vi "auto_alignment_v2.vi"(0 "meter-visa":refnum<visa-resource-name>, 1 "xStart":dbl=264.0 format="%#_13g", 2 "yStart":dbl=123.0 format="%#_13g", 3 "NM-params":T1={"alpha"=1.0, "gamma"=2.0, "rho"=0.5, "sigma"=0.5, "simplex L"=0.5}, 5 "PD Values":cluster{"PD1":dbl, "PD2":dbl, "PD3":dbl}, 6 "F=cRIO":bool, 7 "stage-refs":T2, 9 "meter-error-in":errorcluster, 11 "stage-error-in":errorcluster, 12 "trial #":i32, 13 "path-in":path=path "C:/Users/hpDIRC/Desktop/Tyler/t3.csv") -> (4 "Optimized Location":dbl[](array[numeric]), 8 "squared_error":dbl, 10 "meter-error-out":errorcluster, 14 "run time (min)":dbl, 15 "stage-error-out":errorcluster)   [LabVIEW 2024]
uses:
  O:/DSG/Tyler/EIC/DIRC/daq/automated/Thorlabs.MotionControl.IntegratedStepperMotorsCLI.dll
  Thorlabs.MotionControl.IntegratedStepperMotorsCLI.dll
  O:/DSG/Tyler/EIC/DIRC/daq/automated/Thorlabs.MotionControl.Benchtop.StepperMotorCLI.dll
  Thorlabs.MotionControl.Benchtop.StepperMotorCLI.dll
  5b59031f-b1ff-41af-80a7-e72a33ebffa1.vi
  <vilib>/Array/Sort 2D Array - Pop Stack.vi
  <vilib>/Array/Sort 2D Array - Push Stack.vi
  5b59031f-b1ff-41af-80a7-e72a33ebffa1.vi/269d4b3b-47f5-49e3-8884-44851e4dd9d5.vi
  5b59031f-b1ff-41af-80a7-e72a33ebffa1.vi/6d99389c-673d-4efb-bf33-19b32bcf4cf8.vi
  <vilib>/Analysis/NI_AALBase.lvlib
panel:
  in  "nSamples":dbl=10.0 caption="# Samples"
  in  "simplex-limit":dbl=1e-06 caption="Simplex Length Convergence Goal" format="%#_13g"
  in  "value-limit":dbl=0.04 caption="Value Convergence Goal" format="%#_13g"
  out "Pts Tested":dbl[][](array[numeric])
  out "x_c":dbl[](array[numeric])
  out "x_e":dbl[](array[numeric])
  out "x_r":dbl[](array[numeric])
  out "x_o":dbl[](array[numeric])
  out "iterations timeout":bool
  out "simplex converge":bool
  out "value converge":bool
  out "simplex leg lengths":dbl[](array[numeric])
  in  "stop":bool
  # "centroid"
  # "reflection point"
  # "expansion point"
  # "contraction point"
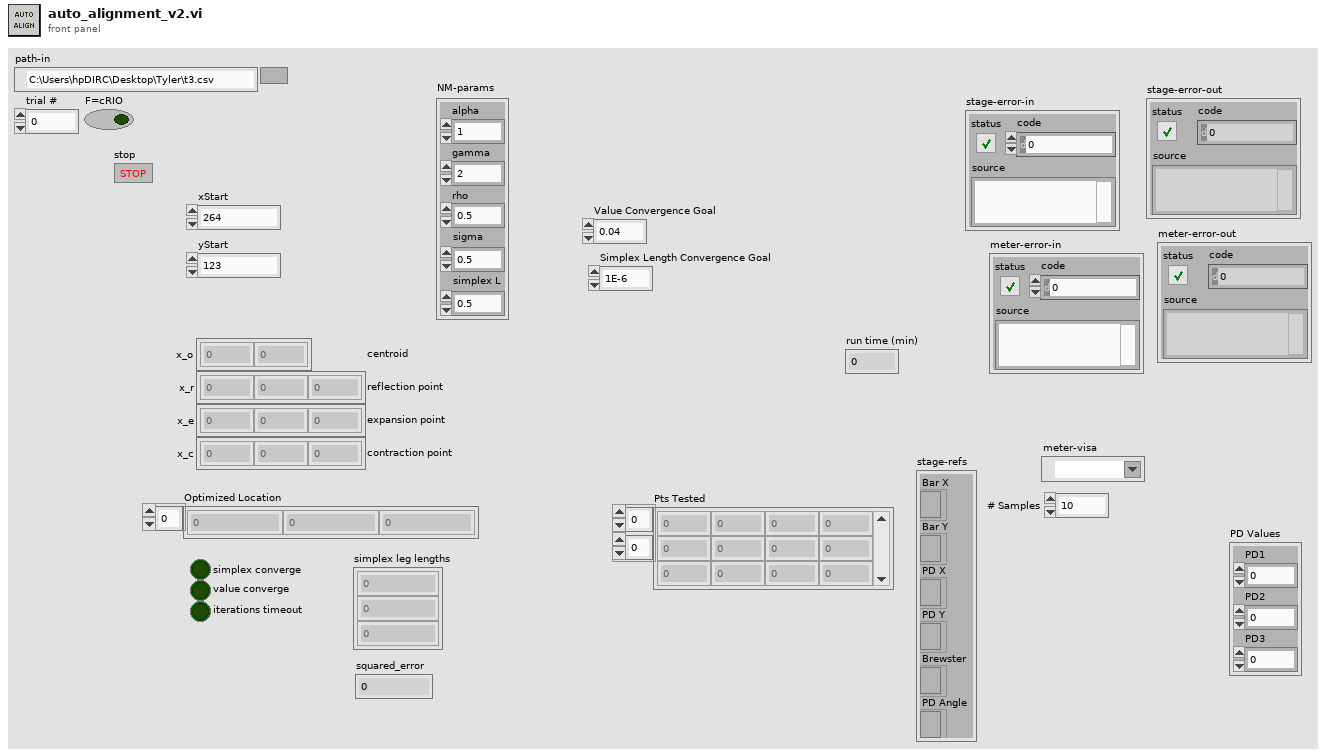
[diagram p1: front panel]
types:
  T1 = cluster{"alpha":dbl, "gamma":dbl, "rho":dbl, "sigma":dbl, "simplex L":dbl}
  T2 = cluster{"Bar X":refnum<k24>, "Bar Y":refnum<k24>, "PD X":refnum<k24>, "PD Y":refnum<k24>, "Brewster":refnum<k24>, "PD Angle":refnum<k24>}
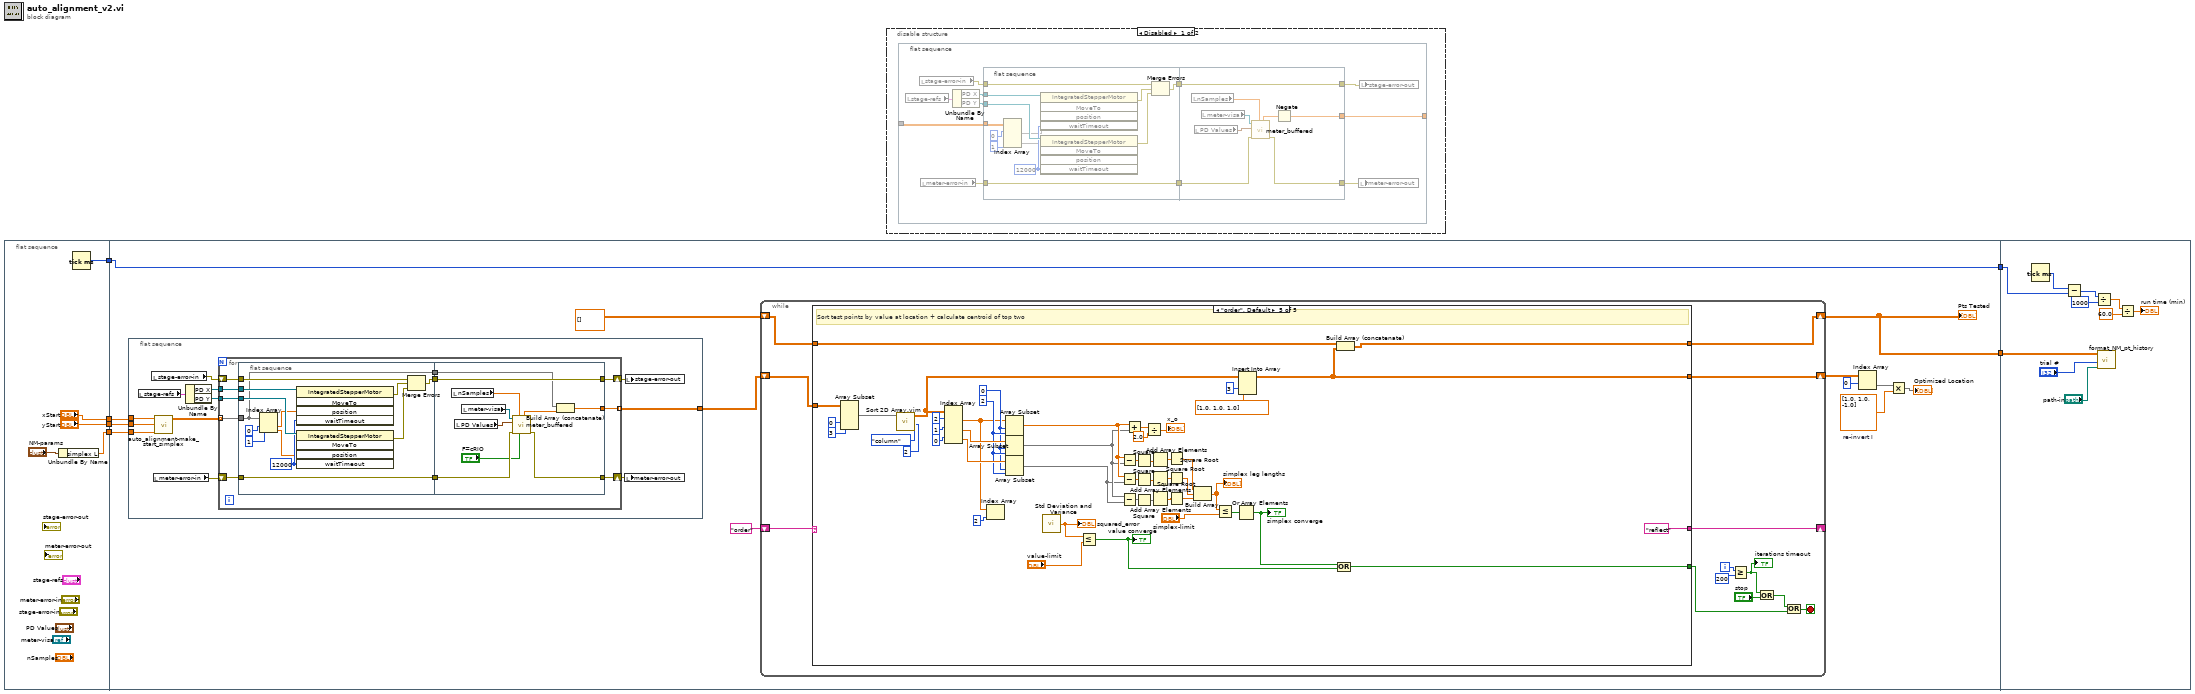
[diagram p0: block diagram]
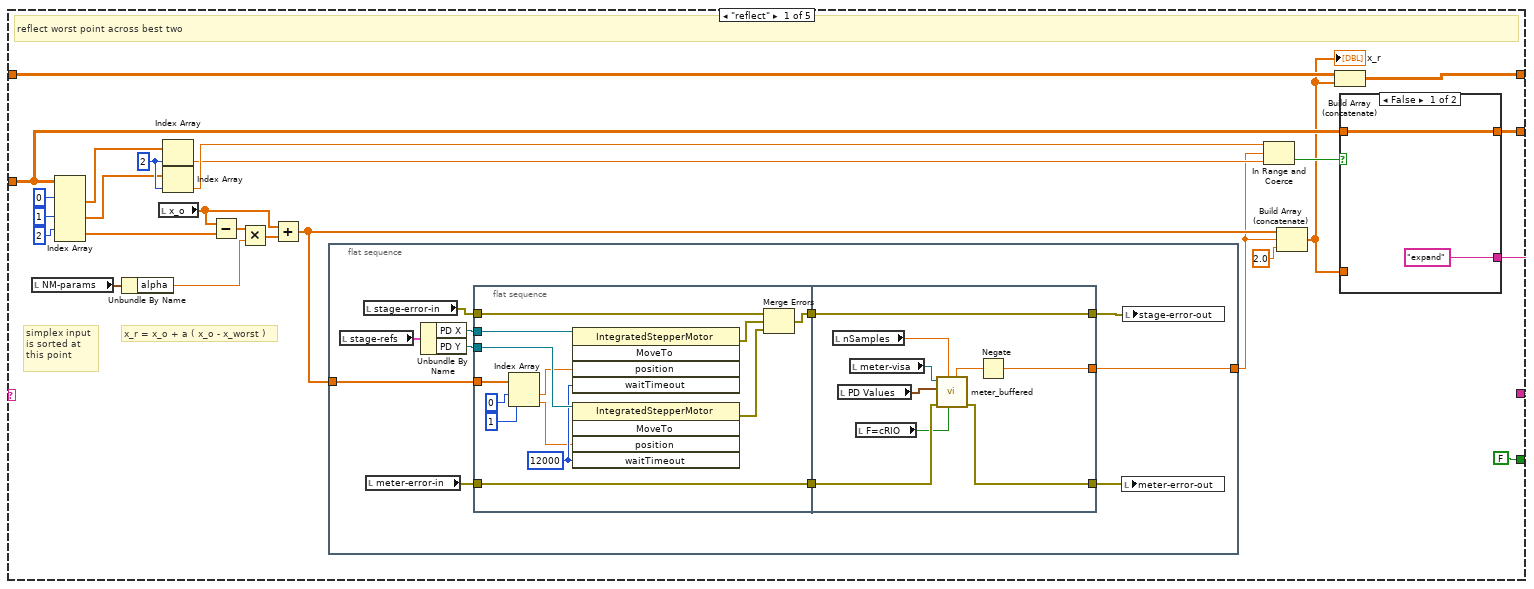
[diagram p3: hidden frame]
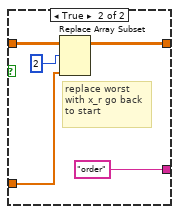
[diagram p4: hidden frame]
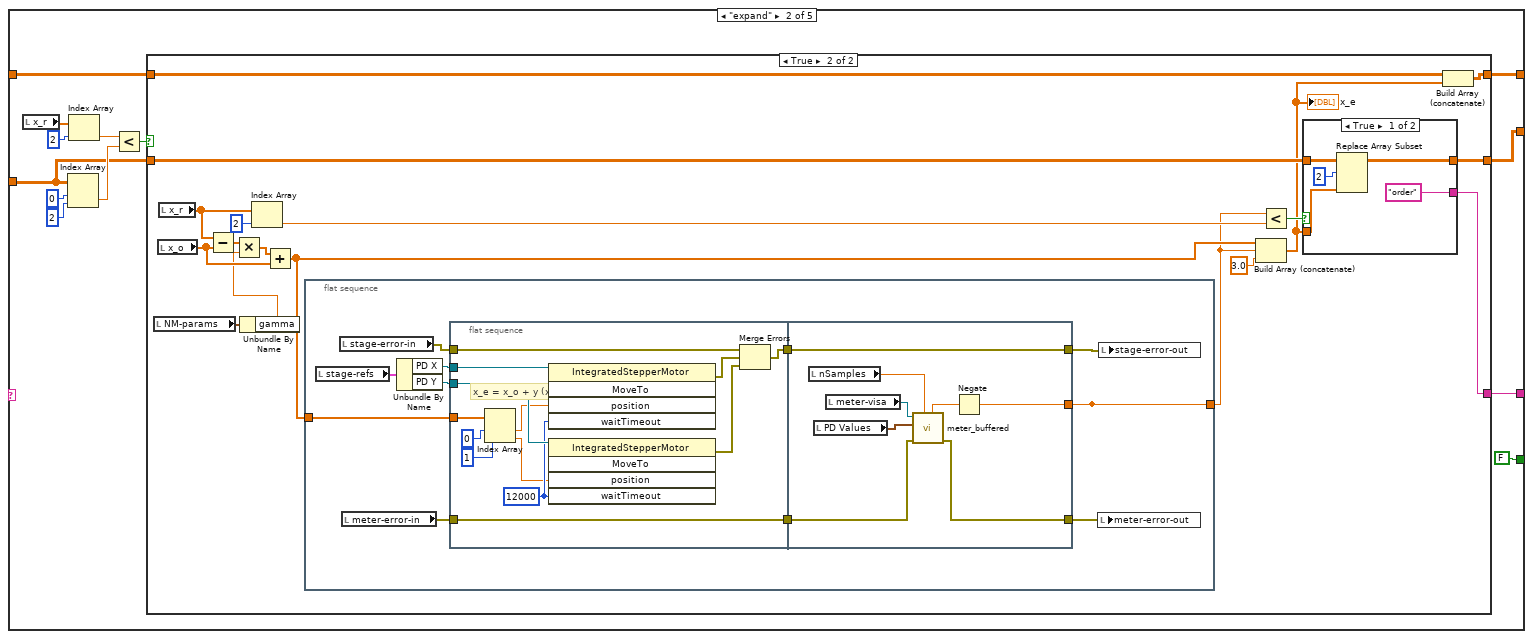
[diagram p5: hidden frame]
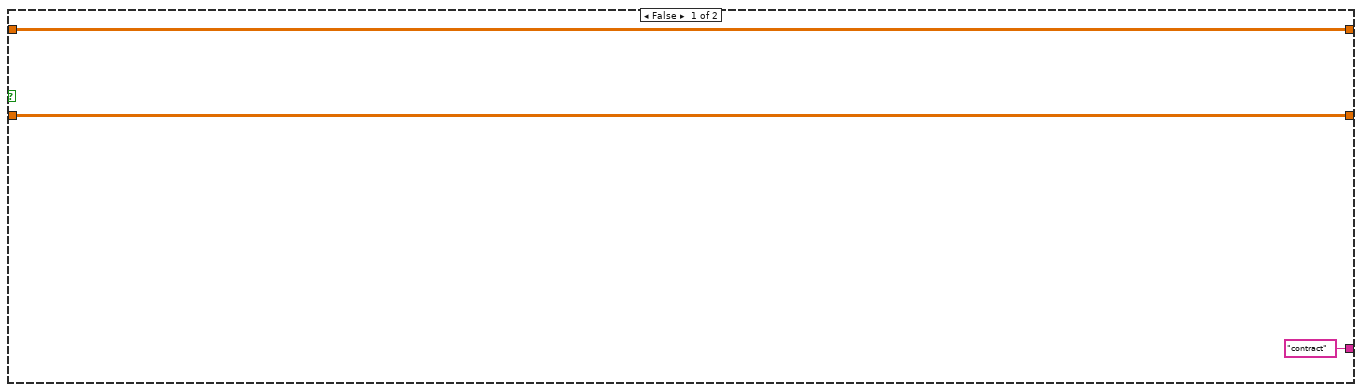
[diagram p6: hidden frame]
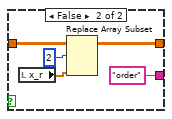
[diagram p7: hidden frame]
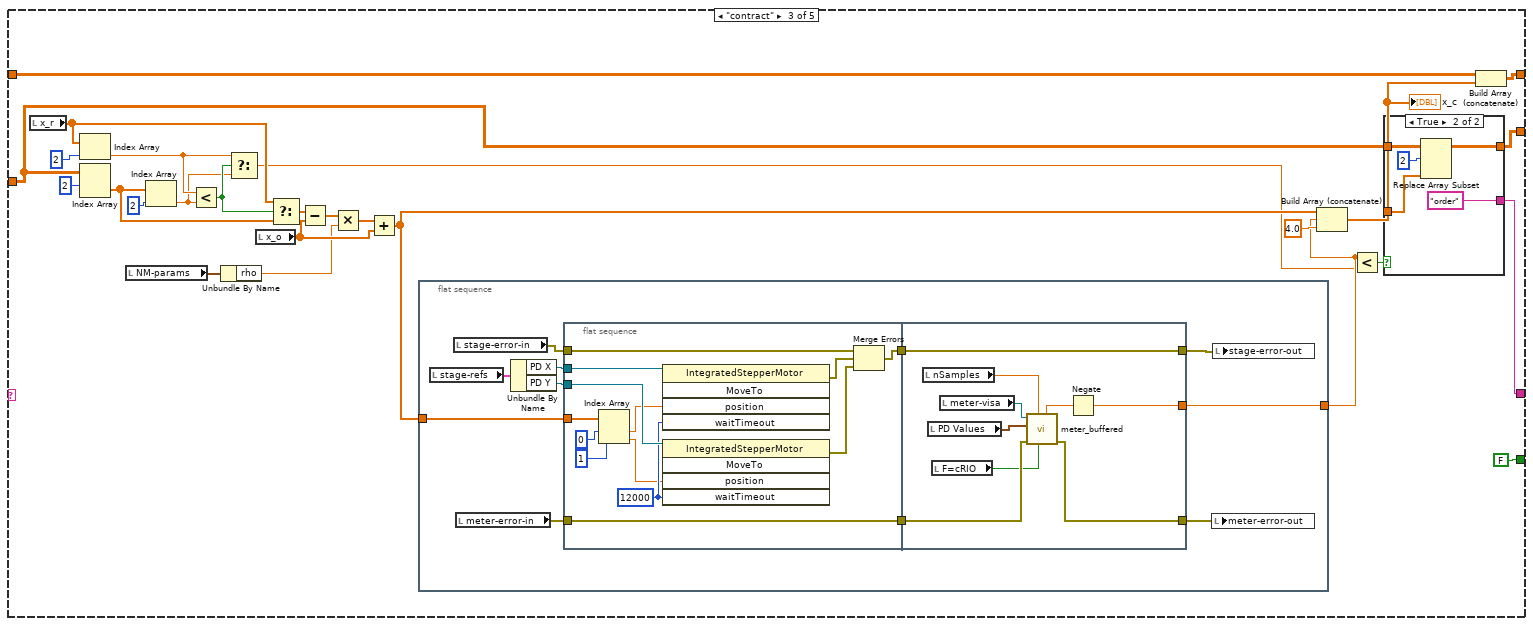
[diagram p8: hidden frame]
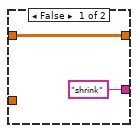
[diagram p9: hidden frame]
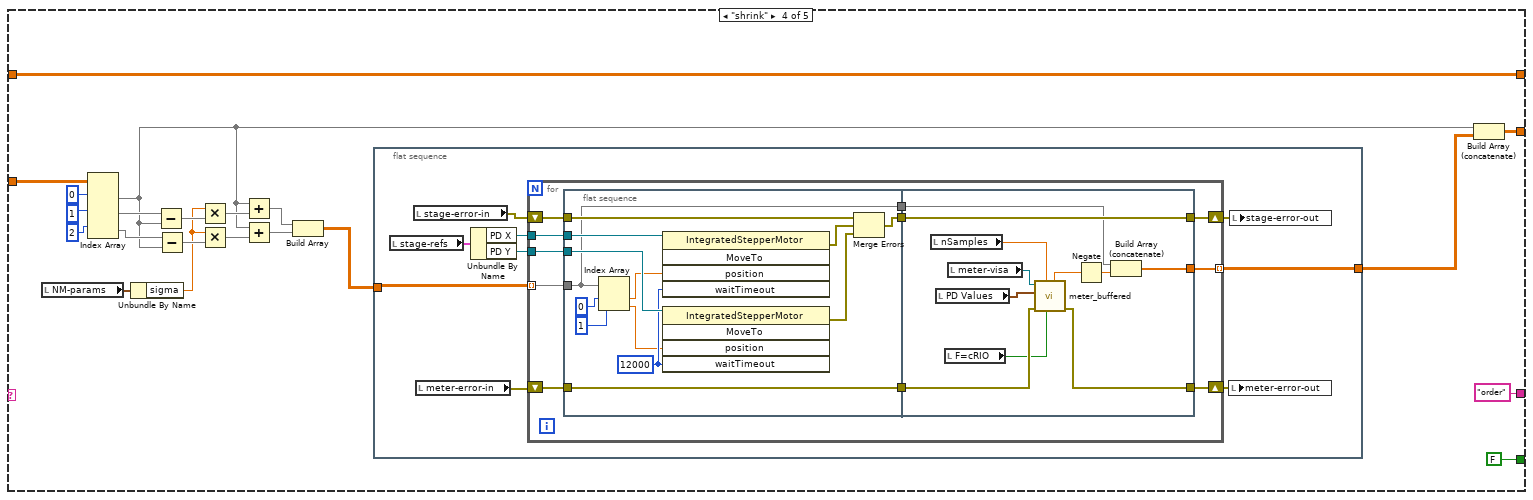
[diagram p10: hidden frame]
diagram:
  n1 = flat-sequence {
    tunnel: [w11] -> w5
    tunnel: ["yStart"] -> w3
    tunnel: ["xStart"] -> w2
    tunnel: [w7] -> w1
    tunnel: [w22] -> w6
    tunnel: w5 -> [w21]
    tunnel: [w21] -> w4
    tunnel: w3 -> [w13]
    tunnel: w2 -> [w14]
    tunnel: w1 -> [w12]
    tunnel: w6 -> [w411]
    tunnel: w4 -> [w409]
    frame #0 {
      n2 = Unbundle By Name("NM-params") -> ("simplex L"=w7:dbl)
      n3 = Tick Count (ms)() -> (millisecond timer value=w11:u32)
    }
    frame #1 {
      w16 = dbl[] [1.0, 1.0, -1.0]  # re-invert I
      n4 = flat-sequence {
        tunnel: [w33] -> w15
        tunnel: w13 -> [w32]
        tunnel: w14 -> [w31]
        tunnel: w12 -> [w25]
        frame #0 {
          n5 = local read "stage-refs"() -> (w27:T2)
          n6 = local read "stage-error-in"() -> (w28:errorcluster)
          n7 = local read "meter-error-in"() -> (w26:errorcluster)
          n8 = call "auto_alignment-make_start_simplex.vi"("L"=w25, "yStart"=w32, "xStart"=w31) -> ("Array"=w34:dbl[][])  [unwired: 8 in]
          n9 = Unbundle By Name(w27) -> ("PD X"=w36:refnum<k24>, "PD Y"=w35:refnum<k24>)
          n10 = for {
            tunnel: w36 -> [w47]
            tunnel: w35 -> [w46]
            tunnel: w34 -> [w43] mode=indexing
            shift-right: [w41] -> w29
            shift-left: w28 -> [w45]
            tunnel: [w44] -> w33 mode=indexing
            shift-right: [w42] -> w30
            shift-left: w26 -> [w40]
            n11 = flat-sequence {
              tunnel: w47 -> [w58]
              tunnel: w46 -> [w57]
              tunnel: w45 -> [w51]
              tunnel: w43 -> [w49]
              tunnel: w40 -> [w48]
              tunnel: [w50] -> w39
              tunnel: [w49] -> w38
              tunnel: [w48] -> w37
              tunnel: [w70] -> w41
              tunnel: [w66] -> w42
              tunnel: [w69] -> w44
              tunnel: w39 -> [w70]
              tunnel: w38 -> [w68]
              tunnel: w37 -> [w67]
              frame #0 {
                w56 = 12000 ("waitTimeout")
                n12 = Index Array(array=w49, index #1=0 ("index"), index #2=1 ("index")) -> (element #1=w53:dbl, element #2=w52:dbl)
                n13 = invoke class="IntegratedStepperMotor" method="MoveTo"(reference=w58, "position"=w53, "waitTimeout"=w56) -> (error out=w60:errorcluster)  [unwired: 2 in, 4 out]
                n14 = invoke class="IntegratedStepperMotor" method="MoveTo"(reference=w57, "position"=w52, "waitTimeout"=w56) -> (error out=w59:errorcluster)  [unwired: 2 in, 4 out]
                n15 = Merge Errors(w51, w60, w59) -> (w50:errorcluster)
              }
              frame #1 {
                n16 = local read "nSamples"() -> (w65:dbl)
                n17 = local read "PD Values"() -> (w63:cluster{"PD1":dbl, "PD2":dbl, "PD3":dbl})
                n18 = local read "meter-visa"() -> (w64:refnum<visa-resource-name>)
                n19 = call "meter_buffered.vi"("F=cRIO"="F=cRIO", "Samples"=w65, "error in"=w67, "PD ranges"=w63, "meter-VISA"=w64) -> ("error out"=w66:errorcluster, "iCorr"=w61:dbl)  [unwired: 2 in, 3 out]
                n20 = Build Array (concatenate)(w68, w61) -> (w69:dbl[])
              }
            }
          }
          n21 = local write "meter-error-out"(w30) -> ()
          n22 = local write "stage-error-out"(w29) -> ()
        }
      }
      n23 = while {
        shift-right: [w81] -> w20
        shift-left: w15 -> [w80]
        shift-right: [w82] -> _
        shift-left: "order" -> [w83]
        shift-right: [w78] -> w22
        shift-left: dbl[][] [] -> [w79]
        i -> [w74]
        stop <- w72 stop-if-true
        n24 = case shown="\"order\", Default" w83 {
          tunnel: w80 -> [w94 w154 w237 w310 w395]
          tunnel: [FALSE FALSE FALSE FALSE w376] -> w76
          tunnel: [w93 w153 w238 w299 w369] -> w81
          tunnel: [w95 w152 w239 "order" "reflect"] -> w82
          tunnel: w79 -> [w91 w150 w233 w297 w368]
          tunnel: [w90 w149 w232 w297 w373] -> w78
          frame "reflect" {
            w102 = 2 ("index")
            # "simplex input\nis sorted at\nthis point"
            # "x_r = x_o + a ( x_o - x_worst )"
            # "reflect worst point across best two"
            n25 = local read "NM-params"() -> (w85:T1)
            n26 = Index Array(array=w94, index (row) #1=0 ("index (row)"), index (row) #2=1 ("index (row)"), index (row) #3=2 ("index (row)")) -> (element #1=w101:dbl[], element #2=w100:dbl[], element #3=w103:dbl[])  [unwired: 3 in]
            n27 = Unbundle By Name(w85) -> ("alpha"=w84:dbl)
            n28 = local read "x_o"() -> (w96:dbl[])
            n29 = Index Array(array=w101, index=w102) -> (element=w98:dbl)
            n30 = Index Array(array=w100, index=w102) -> (element=w99:dbl)
            n31 = Subtract(x=w96, y=w103) -> (x-y=w107:dbl[])
            n32 = Multiply(x=w107, y=w84) -> (x*y=w106:dbl[])
            n33 = Add(x=w96, y=w106) -> (x+y=w87:dbl[])
            n34 = flat-sequence {
              tunnel: [w109] -> w86
              tunnel: w87 -> [w110]
              frame #0 {
                n35 = local read "stage-refs"() -> (w114:T2)
                n36 = local read "stage-error-in"() -> (w115:errorcluster)
                n37 = local read "meter-error-in"() -> (w113:errorcluster)
                n38 = Unbundle By Name(w114) -> ("PD X"=w119:refnum<k24>, "PD Y"=w118:refnum<k24>)
                n39 = flat-sequence {
                  tunnel: w119 -> [w130]
                  tunnel: w118 -> [w129]
                  tunnel: w115 -> [w123]
                  tunnel: w110 -> [w121]
                  tunnel: w113 -> [w120]
                  tunnel: [w122] -> w112
                  tunnel: [w120] -> w111
                  tunnel: [w141] -> w116
                  tunnel: [w138] -> w117
                  tunnel: [w134] -> w109
                  tunnel: w112 -> [w141]
                  tunnel: w111 -> [w139]
                  frame #0 {
                    w128 = 12000 ("waitTimeout")
                    n40 = Index Array(array=w121, index #1=0 ("index"), index #2=1 ("index")) -> (element #1=w125:dbl, element #2=w124:dbl)
                    n41 = invoke class="IntegratedStepperMotor" method="MoveTo"(reference=w130, "position"=w125, "waitTimeout"=w128) -> (error out=w132:errorcluster)  [unwired: 2 in, 4 out]
                    n42 = invoke class="IntegratedStepperMotor" method="MoveTo"(reference=w129, "position"=w124, "waitTimeout"=w128) -> (error out=w131:errorcluster)  [unwired: 2 in, 4 out]
                    n43 = Merge Errors(w123, w132, w131) -> (w122:errorcluster)
                  }
                  frame #1 {
                    n44 = local read "nSamples"() -> (w137:dbl)
                    n45 = local read "PD Values"() -> (w135:cluster{"PD1":dbl, "PD2":dbl, "PD3":dbl})
                    n46 = local read "meter-visa"() -> (w136:refnum<visa-resource-name>)
                    n47 = local read "F=cRIO"() -> (w133:bool)
                    n48 = call "meter_buffered.vi"("F=cRIO"=w133, "Samples"=w137, "error in"=w139, "PD ranges"=w135, "meter-VISA"=w136) -> ("error out"=w138:errorcluster, "iCorr"=w140:dbl)  [unwired: 2 in, 3 out]
                    n49 = Negate(x=w140) -> (-x=w134:dbl)
                  }
                }
                n50 = local write "meter-error-out"(w117) -> ()
                n51 = local write "stage-error-out"(w116) -> ()
              }
            }
            n52 = In Range and Coerce(upper limit=w99, x=w86, lower limit=w98) -> (In Range?=w97:bool)  [unwired: 1 out]
            n53 = Build Array (concatenate)(w87, w86, 2.0) -> (w89:dbl[])
            "x_r" <- w89
            n54 = Build Array (concatenate)(w91, w89) -> (w90:dbl[][])
            n55 = case shown="False" w97 {
              tunnel: ["expand" "order"] -> w95
              tunnel: w94 -> [w142 w148]
              tunnel: [w142 w145] -> w93
              tunnel: w89 -> [_ w146]
              frame False {
              }
              frame True {
                # "replace worst \nwith x_r go back\nto start"
                n56 = Replace Array Subset(array=w148, new element=w146, index (row)=2) -> (w145:dbl[][])  [unwired: 1 in]
              }
            }
          }
          frame "expand" {
            n57 = local read "x_r"() -> (w159:dbl[])
            n58 = Index Array(array=w154, index (row)=0, index (col)=2 ("disabled index (col)")) -> (element=w157:dbl)
            n59 = Index Array(array=w159, index=2) -> (element=w156:dbl)
            n60 = Less?(x=w156, y=w157) -> (x < y?=w155:bool)
            n61 = case shown="True" w155 {
              tunnel: w154 -> [w164 w175]
              tunnel: [w164 w174] -> w153
              tunnel: ["contract" w173] -> w152
              tunnel: w150 -> [w162 w172]
              tunnel: [w162 w171] -> w149
              frame False {
              }
              frame True {
                # "x_e = x_o + y (x _r - x _o)"
                n62 = local read "NM-params"() -> (w166:T1)
                n63 = local read "x_o"() -> (w180:dbl[])
                n64 = local read "x_r"() -> (w179:dbl[])
                n65 = Subtract(x=w179, y=w180) -> (x-y=w182:dbl[])
                n66 = Unbundle By Name(w166) -> ("gamma"=w165:dbl)
                n67 = Multiply(x=w182, y=w165) -> (x*y=w181:dbl[])
                n68 = Index Array(array=w179, index=2) -> (element=w177:dbl)
                n69 = Add(x=w181, y=w180) -> (x+y=w168:dbl[])
                n70 = flat-sequence {
                  tunnel: [w183] -> _
                  tunnel: w168 -> [w184]
                  tunnel: [w183] -> w167
                  frame #0 {
                    n71 = local read "stage-refs"() -> (w188:T2)
                    n72 = local read "stage-error-in"() -> (w189:errorcluster)
                    n73 = local read "meter-error-in"() -> (w187:errorcluster)
                    n74 = Unbundle By Name(w188) -> ("PD X"=w193:refnum<k24>, "PD Y"=w192:refnum<k24>)
                    n75 = flat-sequence {
                      tunnel: w193 -> [w204]
                      tunnel: w192 -> [w203]
                      tunnel: w189 -> [w197]
                      tunnel: w184 -> [w195]
                      tunnel: w187 -> [w194]
                      tunnel: [w196] -> w186
                      tunnel: [w194] -> w185
                      tunnel: [w214] -> w190
                      tunnel: [w211] -> w191
                      tunnel: [w207] -> w183
                      tunnel: w186 -> [w214]
                      tunnel: w185 -> [w212]
                      frame #0 {
                        w202 = 12000 ("waitTimeout")
                        n76 = Index Array(array=w195, index #1=0 ("index"), index #2=1 ("index")) -> (element #1=w199:dbl, element #2=w198:dbl)
                        n77 = invoke class="IntegratedStepperMotor" method="MoveTo"(reference=w204, "position"=w199, "waitTimeout"=w202) -> (error out=w206:errorcluster)  [unwired: 2 in, 4 out]
                        n78 = invoke class="IntegratedStepperMotor" method="MoveTo"(reference=w203, "position"=w198, "waitTimeout"=w202) -> (error out=w205:errorcluster)  [unwired: 2 in, 4 out]
                        n79 = Merge Errors(w197, w206, w205) -> (w196:errorcluster)
                      }
                      frame #1 {
                        n80 = local read "nSamples"() -> (w210:dbl)
                        n81 = local read "PD Values"() -> (w208:cluster{"PD1":dbl, "PD2":dbl, "PD3":dbl})
                        n82 = local read "meter-visa"() -> (w209:refnum<visa-resource-name>)
                        n83 = call "meter_buffered.vi"("Samples"=w210, "error in"=w212, "PD ranges"=w208, "meter-VISA"=w209) -> ("error out"=w211:errorcluster, "iCorr"=w213:dbl)  [unwired: 3 in, 3 out]
                        n84 = Negate(x=w213) -> (-x=w207:dbl)
                      }
                    }
                    n85 = local write "meter-error-out"(w191) -> ()
                    n86 = local write "stage-error-out"(w190) -> ()
                  }
                }
                n87 = Build Array (concatenate)(w168, w167, 3.0) -> (w170:dbl[])
                "x_e" <- w170
                n88 = Less?(x=w167, y=w177) -> (x < y?=w176:bool)
                n89 = case shown="True" w176 {
                  tunnel: w175 -> [w218 w223]
                  tunnel: w170 -> [w217 _]
                  tunnel: [w216 w222] -> w174
                  tunnel: ["order" "order"] -> w173
                  frame True {
                    n90 = Replace Array Subset(array=w218, new element=w217, index (row)=2) -> (w216:dbl[][])  [unwired: 1 in]
                  }
                  frame False {
                    n91 = local read "x_r"() -> (w220:dbl[])
                    n92 = Replace Array Subset(array=w223, new element=w220, index (row)=2) -> (w222:dbl[][])  [unwired: 1 in]
                  }
                }
                n93 = Build Array (concatenate)(w172, w170) -> (w171:dbl[][])
              }
            }
          }
          frame "contract" {
            n94 = local read "x_r"() -> (w247:dbl[])
            n95 = Index Array(array=w247, index=2) -> (element=w242:dbl)
            n96 = Index Array(array=w237, index (row)=2) -> (element=w246:dbl[])  [unwired: 1 in]
            n97 = local read "NM-params"() -> (w227:T1)
            n98 = Index Array(array=w246, index=2) -> (element=w241:dbl)
            n99 = Less?(x=w242, y=w241) -> (x < y?=w243:bool)
            n100 = Unbundle By Name(w227) -> ("rho"=w226:dbl)
            n101 = Select(t=w242, s=w243, f=w241) -> (s? t:f=w225:dbl)
            n102 = local read "x_o"() -> (w235:dbl[])
            n103 = Select(t=w247, s=w243, f=w246) -> (s? t:f=w245:dbl[])
            n104 = Subtract(x=w245, y=w235) -> (x-y=w244:dbl[])
            n105 = Multiply(x=w244, y=w226) -> (x*y=w236:dbl[])
            n106 = Add(x=w236, y=w235) -> (x+y=w229:dbl[])
            n107 = flat-sequence {
              tunnel: [w259] -> w228
              tunnel: w229 -> [w251]
              frame #0 {
                n108 = local read "stage-refs"() -> (w255:T2)
                n109 = local read "stage-error-in"() -> (w256:errorcluster)
                n110 = local read "meter-error-in"() -> (w254:errorcluster)
                n111 = Unbundle By Name(w255) -> ("PD X"=w261:refnum<k24>, "PD Y"=w260:refnum<k24>)
                n112 = flat-sequence {
                  tunnel: w261 -> [w272]
                  tunnel: w260 -> [w271]
                  tunnel: w256 -> [w265]
                  tunnel: w251 -> [w263]
                  tunnel: w254 -> [w262]
                  tunnel: [w264] -> w253
                  tunnel: [w262] -> w252
                  tunnel: [w283] -> w257
                  tunnel: [w280] -> w258
                  tunnel: [w276] -> w259
                  tunnel: w253 -> [w283]
                  tunnel: w252 -> [w281]
                  frame #0 {
                    w270 = 12000 ("waitTimeout")
                    n113 = Index Array(array=w263, index #1=0 ("index"), index #2=1 ("index")) -> (element #1=w267:dbl, element #2=w266:dbl)
                    n114 = invoke class="IntegratedStepperMotor" method="MoveTo"(reference=w272, "position"=w267, "waitTimeout"=w270) -> (error out=w274:errorcluster)  [unwired: 2 in, 4 out]
                    n115 = invoke class="IntegratedStepperMotor" method="MoveTo"(reference=w271, "position"=w266, "waitTimeout"=w270) -> (error out=w273:errorcluster)  [unwired: 2 in, 4 out]
                    n116 = Merge Errors(w265, w274, w273) -> (w264:errorcluster)
                  }
                  frame #1 {
                    n117 = local read "nSamples"() -> (w279:dbl)
                    n118 = local read "PD Values"() -> (w277:cluster{"PD1":dbl, "PD2":dbl, "PD3":dbl})
                    n119 = local read "F=cRIO"() -> (w275:bool)
                    n120 = local read "meter-visa"() -> (w278:refnum<visa-resource-name>)
                    n121 = call "meter_buffered.vi"("F=cRIO"=w275, "Samples"=w279, "error in"=w281, "PD ranges"=w277, "meter-VISA"=w278) -> ("error out"=w280:errorcluster, "iCorr"=w282:dbl)  [unwired: 2 in, 3 out]
                    n122 = Negate(x=w282) -> (-x=w276:dbl)
                  }
                }
                n123 = local write "meter-error-out"(w258) -> ()
                n124 = local write "stage-error-out"(w257) -> ()
              }
            }
            n125 = Build Array (concatenate)(w229, w228, 4.0 ("array")) -> (w231:dbl[])
            "x_c" <- w231
            n126 = Less?(x=w228, y=w225) -> (x < y?=w240:bool)
            n127 = case shown="True" w240 {
              tunnel: ["shrink" "order"] -> w239
              tunnel: [w284 w286] -> w238
              tunnel: w237 -> [w284 w288]
              tunnel: w231 -> [_ w287]
              frame False {
              }
              frame True {
                n128 = Replace Array Subset(array=w288, new element=w287, index (row)=2) -> (w286:dbl[][])  [unwired: 1 in]
              }
            }
            n129 = Build Array (concatenate)(w233, w231) -> (w232:dbl[][])
          }
          frame "shrink" {
            n130 = local read "NM-params"() -> (w292:T1)
            n131 = Index Array(array=w310, index (row) #1=0 ("index (row)"), index (row) #2=1 ("index (row)"), index (row) #3=2 ("index (row)")) -> (element #1=w300:dbl[], element #2=w306:dbl[], element #3=w305:dbl[])  [unwired: 3 in]
            n132 = Unbundle By Name(w292) -> ("sigma"=w291:dbl)
            n133 = Subtract(x=w306, y=w300) -> (x-y=w303:dbl[])
            n134 = Subtract(x=w305, y=w300) -> (x-y=w304:dbl[])
            n135 = Multiply(x=w291, y=w303) -> (x*y=w302:dbl[])
            n136 = Multiply(x=w291, y=w304) -> (x*y=w301:dbl[])
            n137 = Add(x=w300, y=w302) -> (x+y=w296:dbl[])
            n138 = Add(x=w300, y=w301) -> (x+y=w295:dbl[])
            n139 = Build Array(w296, w295) -> (w294:dbl[][])
            n140 = flat-sequence {
              tunnel: [w318] -> w293
              tunnel: w294 -> [w312]
              frame #0 {
                n141 = local read "stage-refs"() -> (w314:T2)
                n142 = local read "stage-error-in"() -> (w315:errorcluster)
                n143 = local read "meter-error-in"() -> (w313:errorcluster)
                n144 = Unbundle By Name(w314) -> ("PD X"=w320:refnum<k24>, "PD Y"=w319:refnum<k24>)
                n145 = for {
                  tunnel: w320 -> [w331]
                  tunnel: w319 -> [w330]
                  tunnel: w312 -> [w327] mode=indexing
                  shift-right: [w325] -> w316
                  shift-left: w315 -> [w329]
                  tunnel: [w328] -> w318 mode=indexing
                  shift-right: [w326] -> w317
                  shift-left: w313 -> [w324]
                  n146 = flat-sequence {
                    tunnel: w331 -> [w342]
                    tunnel: w330 -> [w341]
                    tunnel: w329 -> [w335]
                    tunnel: w327 -> [w333]
                    tunnel: w324 -> [w332]
                    tunnel: [w334] -> w323
                    tunnel: [w333] -> w322
                    tunnel: [w332] -> w321
                    tunnel: [w355] -> w325
                    tunnel: [w349] -> w326
                    tunnel: [w352] -> w328
                    tunnel: w323 -> [w355]
                    tunnel: w322 -> [w351]
                    tunnel: w321 -> [w350]
                    frame #0 {
                      w340 = 12000 ("waitTimeout")
                      n147 = Index Array(array=w333, index #1=0 ("index"), index #2=1 ("index")) -> (element #1=w337:dbl, element #2=w336:dbl)
                      n148 = invoke class="IntegratedStepperMotor" method="MoveTo"(reference=w342, "position"=w337, "waitTimeout"=w340) -> (error out=w344:errorcluster)  [unwired: 2 in, 4 out]
                      n149 = invoke class="IntegratedStepperMotor" method="MoveTo"(reference=w341, "position"=w336, "waitTimeout"=w340) -> (error out=w343:errorcluster)  [unwired: 2 in, 4 out]
                      n150 = Merge Errors(w335, w344, w343) -> (w334:errorcluster)
                    }
                    frame #1 {
                      n151 = local read "nSamples"() -> (w348:dbl)
                      n152 = local read "PD Values"() -> (w346:cluster{"PD1":dbl, "PD2":dbl, "PD3":dbl})
                      n153 = local read "F=cRIO"() -> (w345:bool)
                      n154 = local read "meter-visa"() -> (w347:refnum<visa-resource-name>)
                      n155 = call "meter_buffered.vi"("F=cRIO"=w345, "Samples"=w348, "error in"=w350, "PD ranges"=w346, "meter-VISA"=w347) -> ("error out"=w349:errorcluster, "iCorr"=w353:dbl)  [unwired: 2 in, 3 out]
                      n156 = Negate(x=w353) -> (-x=w354:dbl)
                      n157 = Build Array (concatenate)(w351, w354) -> (w352:dbl[])
                    }
                  }
                }
                n158 = local write "meter-error-out"(w317) -> ()
                n159 = local write "stage-error-out"(w316) -> ()
              }
            }
            n160 = Build Array (concatenate)(w300, w293) -> (w299:dbl[][])
          }
          frame "order", Default {
            w359 = 2 ("length")
            w358 = 0 ("index")
            # "Sort test points by value at location + calculate centroid of top two"
            n161 = Array Subset(array=w395, index (col)=0 ("index"), length (col)=3 ("length")) -> (w367:dbl[][])  [unwired: 2 in]
            n162 = call "Sort 2D Array.vim"("index"=2, "dimension to index (column)"=enum16{"column", "row"}."column", "2D array"=w367) -> ("sorted 2D array"=w365:dbl[][])  [unwired: 7 in, 1 out]
            n163 = Index Array(array=w365, index (row) #1=2 ("index (row)"), index (row) #2=1 ("index (row)"), index (row) #3=0 ("index (row)")) -> (element #1=w357:dbl[], element #2=w362:dbl[], element #3=w360:dbl[])  [unwired: 3 in]
            n164 = Index Array(array=w357, index=2) -> ()  [unwired: 1 out]
            n165 = Array Subset(array=w357, index=w358, length=w359) -> (w364:dbl[])
            n166 = Array Subset(array=w362, index=w358, length=w359) -> (w363:dbl[])
            n167 = Array Subset(array=w360, index=w358, length=w359) -> (w361:dbl[])
            n168 = call <vilib>:"Std Deviation and Variance.vi"() -> ("standard deviation"=w372:dbl)  [unwired: 2 in, 2 out]
            "squared_error" <- w372
            n169 = Less Or Equal?(x=w372, y="value-limit") -> (x <= y?=w375:bool)
            "value converge" <- w375
            n170 = Subtract(x=w364, y=w363) -> (x-y=w390:dbl[])
            n171 = Subtract(x=w364, y=w361) -> (x-y=w382:dbl[])
            n172 = Subtract(x=w363, y=w361) -> (x-y=w385:dbl[])
            n173 = Add(x=w364, y=w363) -> (x+y=w393:dbl[])
            n174 = Square(x=w390) -> (x^2=w389:dbl[])
            n175 = Square(x=w382) -> (x^2=w386:dbl[])
            n176 = Square(x=w385) -> (x^2=w384:dbl[])
            n177 = Divide(x=w393, y=2.0) -> (x/y=→"x_o":dbl[])
            n178 = Add Array Elements(numeric array=w389) -> (sum=w388:dbl)
            n179 = Add Array Elements(numeric array=w386) -> (sum=w387:dbl)
            n180 = Add Array Elements(numeric array=w384) -> (sum=w383:dbl)
            n181 = Square Root(x=w388) -> (sqrt(x)=w379:dbl)
            n182 = Square Root(x=w387) -> (sqrt(x)=w380:dbl)
            n183 = Square Root(x=w383) -> (sqrt(x)=w381:dbl)
            n184 = Build Array(w379, w380, w381) -> (w378:dbl[])
            "simplex leg lengths" <- w378
            n185 = Less Or Equal?(x=w378, y="simplex-limit") -> (x <= y?=w377:bool[])
            n186 = Or Array Elements(Boolean array=w377) -> (logical OR=w374:bool)
            "simplex converge" <- w374
            n187 = Insert Into Array(array=w365, index (col)=3 ("disabled index (col)"), new element=dbl[] [1.0, 1.0, 1.0] ("new element/subarray")) -> (w369:dbl[][])  [unwired: 1 in]
            n188 = Build Array (concatenate)(w368, w369) -> (w373:dbl[][])
            n189 = Compound Arithmetic op=OR(w374, w375) -> (w376:bool)
          }
        }
        n190 = Greater Or Equal?(x=w74, y=200) -> (x >= y?=w73:bool)
        "iterations timeout" <- w73
        n191 = Compound Arithmetic op=OR(w73, "stop") -> (w71:bool)
        n192 = Compound Arithmetic op=OR(w71, w76) -> (w72:bool)
      }
      "Pts Tested" <- w22
      n193 = Index Array(array=w20, index (row)=0) -> (element=w17:dbl[])  [unwired: 1 in]
      n194 = Multiply(x=w17, y=w16) -> (x*y=→"Optimized Location":dbl[])
    }
    frame #2 {
      n195 = Tick Count (ms)() -> (millisecond timer value=w410:u32)
      n196 = Subtract(x=w410, y=w409) -> (x-y=w408:u32)
      n197 = Divide(x=w408, y=u32 1000) -> (x/y=w406:dbl)
      n198 = call "format_NM_pt_history.vi"("path-in"="path-in", "trial #"="trial #", "data in"=w411) -> ()  [unwired: 9 in]
      n199 = Divide(x=w406, y=60.0) -> (x/y=→"run time (min)":dbl)
    }
  }
  n200 = disable-structure shown="Disabled" {
    frame Disabled {
      n201 = flat-sequence {
        tunnel: [w422] -> _
        tunnel: [w414] -> _
        frame #0 {
          n202 = local read "stage-refs"() -> (w418:T2)
          n203 = local read "stage-error-in"() -> (w419:errorcluster)
          n204 = local read "meter-error-in"() -> (w417:errorcluster)
          n205 = Unbundle By Name(w418) -> ("PD X"=w424:refnum<k24>, "PD Y"=w423:refnum<k24>)
          n206 = flat-sequence {
            tunnel: w424 -> [w435]
            tunnel: w423 -> [w434]
            tunnel: w419 -> [w428]
            tunnel: [w426] -> w414
            tunnel: w417 -> [w425]
            tunnel: [w427] -> w416
            tunnel: [w425] -> w415
            tunnel: [w445] -> w420
            tunnel: [w442] -> w421
            tunnel: [w438] -> w422
            tunnel: w416 -> [w445]
            tunnel: w415 -> [w443]
            frame #0 {
              w433 = 12000 ("waitTimeout")
              n207 = Index Array(array=w426, index (row) #1=0 ("index"), index (row) #2=1 ("index")) -> (element #1=w430, element #2=w429)  [unwired: 2 in]
              n208 = invoke class="IntegratedStepperMotor" method="MoveTo"(reference=w435, "position"=w430, "waitTimeout"=w433) -> (error out=w437:errorcluster)  [unwired: 2 in, 4 out]
              n209 = invoke class="IntegratedStepperMotor" method="MoveTo"(reference=w434, "position"=w429, "waitTimeout"=w433) -> (error out=w436:errorcluster)  [unwired: 2 in, 4 out]
              n210 = Merge Errors(w428, w437, w436) -> (w427:errorcluster)
            }
            frame #1 {
              n211 = local read "nSamples"() -> (w441:dbl)
              n212 = local read "PD Values"() -> (w439:cluster{"PD1":dbl, "PD2":dbl, "PD3":dbl})
              n213 = local read "meter-visa"() -> (w440:refnum<visa-resource-name>)
              n214 = call "meter_buffered.vi"("Samples"=w441, "error in"=w443, "PD ranges"=w439, "meter-VISA"=w440) -> ("error out"=w442:errorcluster, "iCorr"=w444:dbl)  [unwired: 3 in, 3 out]
              n215 = Negate(x=w444) -> (-x=w438:dbl)
            }
          }
          n216 = local write "meter-error-out"(w421) -> ()
          n217 = local write "stage-error-out"(w420) -> ()
        }
      }
    }
    frame Enabled {
    }
  }
